vi "Set Files Channels Array.vi"(8 "error in (no error)":errorcluster, 11 "Plot in":refnum<class "Plot.lvclass">) -> (0 "error out":errorcluster, 3 "Plot out":refnum<class "Plot.lvclass">)   [LabVIEW 2015, in "Plot.lvclass"]
uses:
  Plot.lvclass
  Plot.lvclass/Plot.ctl
  Read Files.vi
  Write File-group-channel.vi
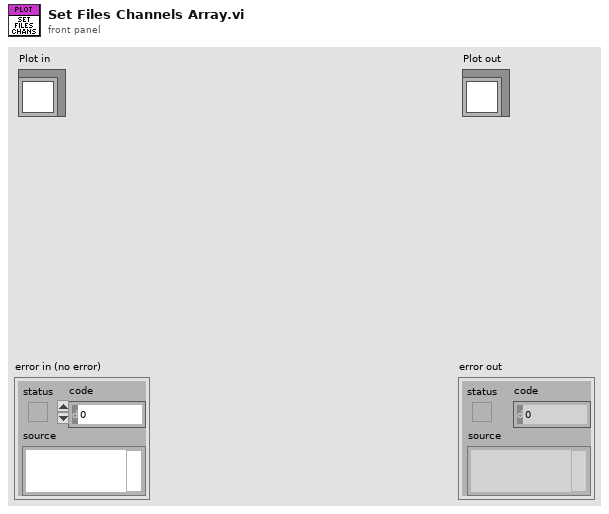
[diagram p1: front panel]
types:
  T1 = typedef "File_Group_Chan_Abbr.ctl" = cluster{"File Path Control":path, "Group":string, "Channel":string, "Abbreviated":string}
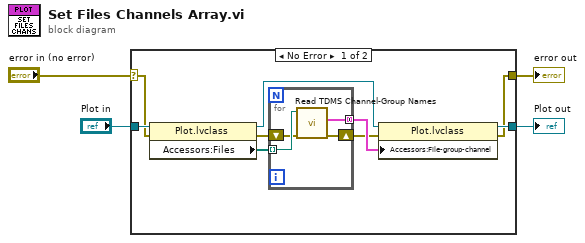
[diagram p0: block diagram]
diagram:
  n1 = case shown="No Error" "error in (no error)" {
    selector: "error in (no error)" -> [w5 w19]
    tunnel: [w6 w19] -> w3
    tunnel: [w10 w18] -> w1
    tunnel: "Plot in" -> [w13 w18]
    frame No Error {
      n2 = property class="Plot.lvclass"(reference=w13, error in=w5) -> (reference out=w12:refnum<class "Plot.lvclass">, error out=w8:errorcluster, "Accessors:Files"=w11:path[])
      n3 = for {
        tunnel: w11 -> [w17] mode=indexing
        tunnel: [w16] -> w9 mode=concatenating
        shift-right: [w14] -> w7
        shift-left: w8 -> [w15]
        n4 = call "Read TDMS Channel-Group Names.vi"("error in"=w15, "File Path Control"=w17) -> ("error out"=w14:errorcluster, "File-group-channel"=w16:T1[])  [unwired: 8 in]
      }
      n5 = property class="Plot.lvclass"(reference=w12, error in=w7, "Accessors:File-group-channel"=w9) -> (reference out=w10:refnum<class "Plot.lvclass">, error out=w6:errorcluster)
    }
    frame Error {
    }
  }
  "error out" <- w3
  "Plot out" <- w1
